vi "Logger.Variant.ReadAll.New.vi"(8 "error in (no error)":errorcluster, 11 "FilePath":path) -> (0 "error out":errorcluster, 1 "Orders 2":cluster{string, string, string, string}[](array[cluster]), 2 "OrdersDetails":T1[](array[typedef]))   [LabVIEW 2016]
uses:
  Sequence/Sequence.Code.SerialFormat.ctl
  Logger.Variant.Sets.ctl
  Station/Station.Changeover.State.vi
  Station/Station.Plate.Properties.ctl
  Drivers/V7310/LowLevel/V7310.Job.Sets.ctl
panel:
  in  "SerialFormat":T4
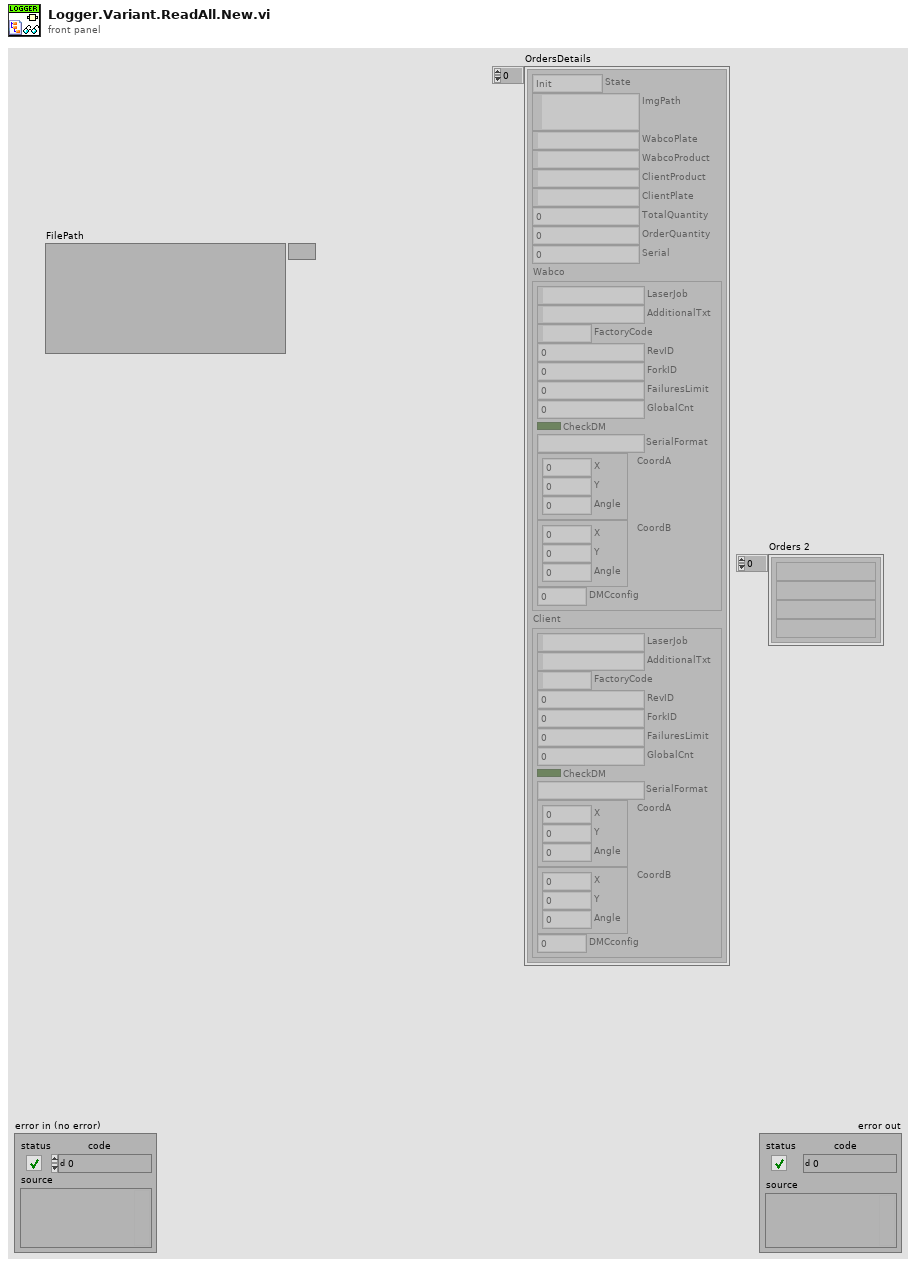
[diagram p1: front panel]
types:
  T1 = typedef "Logger.Variant.Sets.ctl" = cluster{"State":T2, "ImgPath":path, "WabcoPlate":string, "WabcoProduct":string, "ClientProduct":string, "ClientPlate":string, "TotalQuantity":u16, "OrderQuantity":u16, "Serial":i32, "Wabco":T3, "Client":T3}
  T2 = typedef "Station.Changeover.State.vi" = enum16{"Init", "Scaning", "NOK", "Wait for ack", "Ready"}
  T3 = typedef "Station.Plate.Properties.ctl" = cluster{"LaserJob":string, "AdditionalTxt":string, "FactoryCode":string, "RevID":u8, "ForkID":u8, "FailuresLimit":u16, "GlobalCnt":i32, "CheckDM":bool, "SerialFormat":T4, "CoordA":T5, "CoordB":T5, "DMCconfig":i32}
  T4 = typedef "Sequence.Code.SerialFormat.ctl" = enum8{"", "6 dig", "7 dig"}
  T5 = typedef "V7310.Job.Sets.ctl" = cluster{"X":dbl, "Y":dbl, "Angle":dbl}
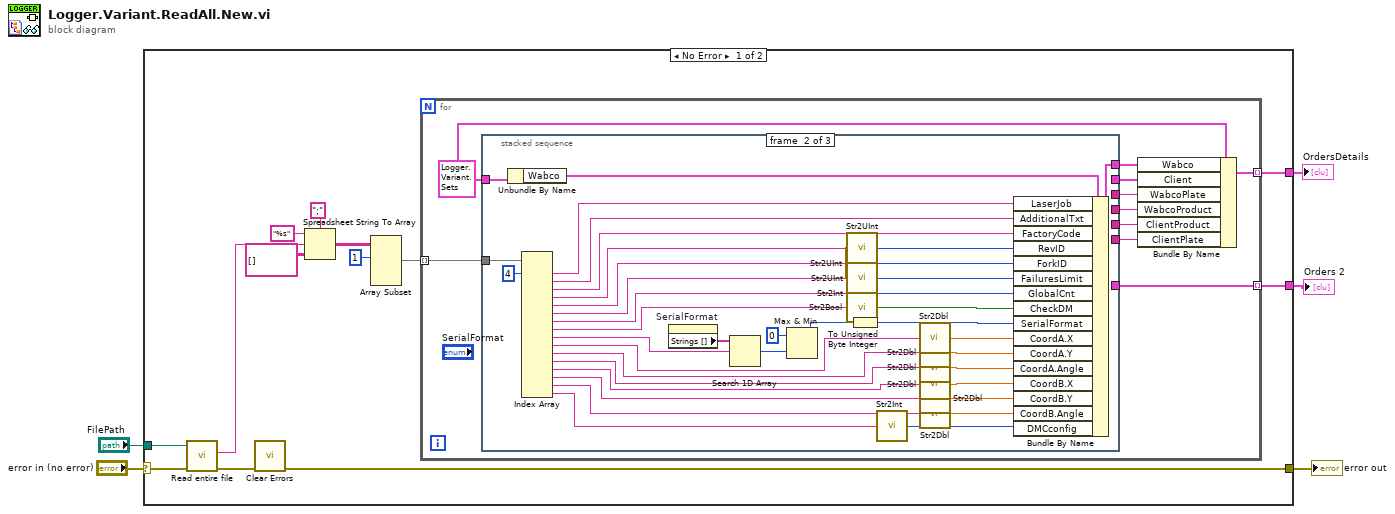
[diagram p0: block diagram]
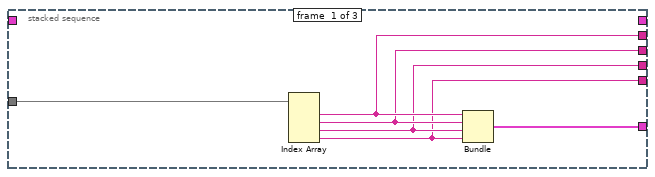
[diagram p2: hidden frame]
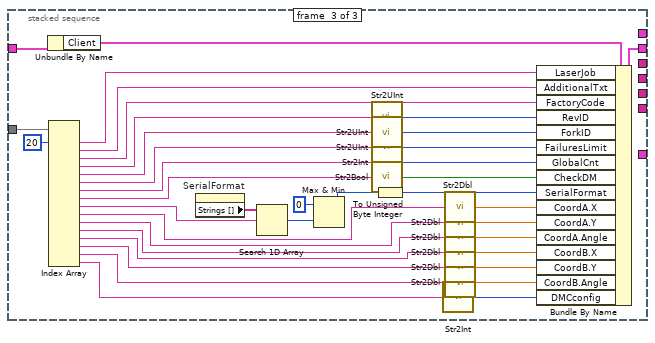
[diagram p3: hidden frame]
diagram:
  n1 = case shown="No Error" "error in (no error)" {
    selector: "error in (no error)" -> [w18 w111]
    tunnel: [w11 w111] -> w4
    tunnel: [w10 _] -> w3
    tunnel: "FilePath" -> [w7 _]
    tunnel: [w6 _] -> w1
    frame No Error {
      n2 = call "Read entire file.vi"("error in"=w18, "file"=w7) -> ("error out"=w12:errorcluster, "contents"=w17:string)  [unwired: 4 in]
      n3 = call <vilib>:"Clear Errors.vi"("error in (no error)"=w12) -> ("error out"=w11:errorcluster)  [unwired: 5 in, 1 out]
      n4 = Spreadsheet String To Array(delimiter (Tab)=";", format string="%s", spreadsheet string=w17, array type (2D Dbl)=string[][] []) -> (array=w9:string[][])
      n5 = Array Subset(array=w9, index (row)=1 ("index")) -> (w8:string[][])  [unwired: 3 in]
      n6 = for {
        tunnel: [w28] -> w10 mode=indexing
        tunnel: w8 -> [w25] mode=indexing
        tunnel: [w19] -> w6 mode=indexing
        w24 = T1 {"State"=enum."Init", "ImgPath"=path "", "WabcoPlate"="", "WabcoProduct"="", "ClientProduct"="", "ClientPlate"="", "TotalQuantity"=0, "OrderQuantity"=0, "Serial"=0, "Wabco"={"LaserJob"="", "AdditionalTxt"="037", "FactoryCode"="", "RevID"=0, "ForkID"=0, "FailuresLimit"=0, "GlobalCnt"=0, "CheckDM"=FALSE, "SerialFormat"=enum."6 dig", "CoordA"={"X"=0.0, "Y"=0.0, "Angle"=0.0}, "CoordB"={"X"=0.0, "Y"=0.0, "Angle"=0.0}, "DMCconfig"=0}, "Client"={"LaserJob"="", "AdditionalTxt"="", "FactoryCode"="037", "RevID"=0, "ForkID"=0, "FailuresLimit"=0, "GlobalCnt"=0, "CheckDM"=FALSE, "SerialFormat"=enum."6 dig", "CoordA"={"X"=0.0, "Y"=0.0, "Angle"=0.0}, "CoordB"={"X"=0.0, "Y"=0.0, "Angle"=0.0}, "DMCconfig"=0}} ("VariantSets in")
        n7 = stacked-sequence {
          tunnel: w25 -> [w34 w70 w108]
          tunnel: w24 -> [_ w40 w88]
          tunnel: [_ w68 _] -> w27
          tunnel: [_ _ w89] -> w26
          tunnel: [w33 _ _] -> w23
          tunnel: [w32 _ _] -> w22
          tunnel: [w31 _ _] -> w21
          tunnel: [w30 _ _] -> w20
          tunnel: [w29 _ _] -> w19
          frame #0 {
            n8 = Index Array(array=w34) -> (element #1=w33:string, element #2=w32:string, element #3=w31:string, element #4=w30:string)  [unwired: 4 in]
            n9 = Bundle(w33, w32, w31, w30) -> (w29:cluster{string, string, string, string})  [unwired: 1 in]
          }
          frame #1 {
            n10 = Unbundle By Name(w40) -> ("Wabco"=w72:T3)
            n11 = Index Array(array=w70, index #1=4 ("index")) -> (element #1=w69:string, element #2=w67:string, element #3=w39:string, element #4=w65:string, element #5=w37:string, element #6=w63:string, element #7=w61:string, element #8=w59:string, element #9=w47:string, element #10=w46:string, element #11=w45:string, element #12=w44:string, element #13=w43:string, element #14=w42:string, element #15=w41:string, element #16=w36:string)  [unwired: 15 in]
            n12 = property on="SerialFormat" class="Enum (strict)"() -> ("Strings []"=w58:string[])  [unwired: 2 in, 2 out]
            n13 = Search 1D Array(1D array=w58, element=w47) -> (index of element=w57:i32)  [unwired: 1 in]
            n14 = Max & Min(x=0, y=w57) -> (max(x,y)=w54:i32)  [unwired: 1 out]
            n15 = call "Str2UInt.vi"("string"=w37) -> ("Numeric"=w38:u32)
            n16 = call "Str2UInt.vi"("string"=w65) -> ("Numeric"=w66:u32)
            n17 = call "Str2UInt.vi"("string"=w63) -> ("Numeric"=w64:u32)
            n18 = call "Str2Int.vi"("string"=w61) -> ("Numeric"=w62:i32)
            n19 = call "Str2Bool.vi"("string"=w59) -> ("Boolean"=w60:bool)
            n20 = To Unsigned Byte Integer(number=w54) -> (unsigned 8bit integer=w55:u8)
            n21 = call "Str2Int.vi"("string"=w36) -> ("Numeric"=w35:i32)
            n22 = call "Str2Dbl.vi"("string"=w46) -> ("Numeric"=w53:dbl)
            n23 = call "Str2Dbl.vi"("string"=w45) -> ("Numeric"=w52:dbl)
            n24 = call "Str2Dbl.vi"("string"=w44) -> ("Numeric"=w51:dbl)
            n25 = call "Str2Dbl.vi"("string"=w43) -> ("Numeric"=w50:dbl)
            n26 = call "Str2Dbl.vi"("string"=w42) -> ("Numeric"=w49:dbl)
            n27 = call "Str2Dbl.vi"("string"=w41) -> ("Numeric"=w48:dbl)
            n28 = Bundle By Name(cluster=w72, "LaserJob"=w69, "AdditionalTxt"=w67, "FactoryCode"=w39, "RevID"=w66, "ForkID"=w38, "FailuresLimit"=w64, "GlobalCnt"=w62, "CheckDM"=w60, "SerialFormat"=w55, "CoordA.X"=w53, "CoordA.Y"=w52, "CoordA.Angle"=w51, "CoordB.X"=w50, "CoordB.Y"=w49, "CoordB.Angle"=w48, "DMCconfig"=w35) -> (w68:T3)
          }
          frame #2 {
            n29 = Unbundle By Name(w88) -> ("Client"=w110:T3)
            n30 = Index Array(array=w108, index #1=20 ("index")) -> (element #1=w107:string, element #2=w106:string, element #3=w105:string, element #4=w103:string, element #5=w102:string, element #6=w100:string, element #7=w98:string, element #8=w96:string, element #9=w90:string, element #10=w85:string, element #11=w84:string, element #12=w83:string, element #13=w86:string, element #14=w87:string, element #15=w82:string, element #16=w74:string)  [unwired: 15 in]
            n31 = property on="SerialFormat" class="Enum (strict)"() -> ("Strings []"=w95:string[])  [unwired: 2 in, 2 out]
            n32 = Search 1D Array(1D array=w95, element=w90) -> (index of element=w94:i32)  [unwired: 1 in]
            n33 = Max & Min(x=0, y=w94) -> (max(x,y)=w91:i32)  [unwired: 1 out]
            n34 = call "Str2UInt.vi"("string"=w103) -> ("Numeric"=w104:u32)
            n35 = call "Str2UInt.vi"("string"=w102) -> ("Numeric"=w75:u32)
            n36 = call "Str2UInt.vi"("string"=w100) -> ("Numeric"=w101:u32)
            n37 = call "Str2Int.vi"("string"=w98) -> ("Numeric"=w99:i32)
            n38 = call "Str2Bool.vi"("string"=w96) -> ("Boolean"=w97:bool)
            n39 = To Unsigned Byte Integer(number=w91) -> (unsigned 8bit integer=w92:u8)
            n40 = call "Str2Int.vi"("string"=w74) -> ("Numeric"=w73:i32)
            n41 = call "Str2Dbl.vi"("string"=w85) -> ("Numeric"=w81:dbl)
            n42 = call "Str2Dbl.vi"("string"=w84) -> ("Numeric"=w80:dbl)
            n43 = call "Str2Dbl.vi"("string"=w83) -> ("Numeric"=w79:dbl)
            n44 = call "Str2Dbl.vi"("string"=w86) -> ("Numeric"=w78:dbl)
            n45 = call "Str2Dbl.vi"("string"=w87) -> ("Numeric"=w77:dbl)
            n46 = call "Str2Dbl.vi"("string"=w82) -> ("Numeric"=w76:dbl)
            n47 = Bundle By Name(cluster=w110, "LaserJob"=w107, "AdditionalTxt"=w106, "FactoryCode"=w105, "RevID"=w104, "ForkID"=w75, "FailuresLimit"=w101, "GlobalCnt"=w99, "CheckDM"=w97, "SerialFormat"=w92, "CoordA.X"=w81, "CoordA.Y"=w80, "CoordA.Angle"=w79, "CoordB.X"=w78, "CoordB.Y"=w77, "CoordB.Angle"=w76, "DMCconfig"=w73) -> (w89:T3)
          }
        }
        n48 = Bundle By Name(cluster=w24, "Wabco"=w27, "Client"=w26, "WabcoPlate"=w23, "WabcoProduct"=w22, "ClientProduct"=w21, "ClientPlate"=w20) -> (w28:T1)
      }
    }
    frame Error {
    }
  }
  "error out" <- w4
  "OrdersDetails" <- w3
  "Orders 2" <- w1
